vi "Add_TF_Ref.vi"(6 "TCP Ref":refnum<k5>, 8 "error in":errorcluster caption="错误输入", 10 "index":i32) -> (0 "error out":errorcluster caption="错误输出")   [LabVIEW 2015]
uses:
  Global/SeverGlobal.vi
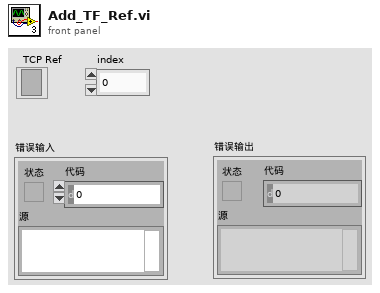
[diagram p1: front panel]
types:
  T1 = cluster{"TCP Ref":refnum<k5>, "Broadcast":refnum<k5>, "TF Ref":refnum<k5>, "IP":string, "port":u16, "userName":string, "passWord":string, "authority":string}[]
  T2 = cluster{"TCP Ref":refnum<k5>, "Broadcast":refnum<k5>, "TF":refnum<k5>, "IP":string, "port":u16, "userName":string, "passWord":string, "authority":string}
  T3 = cluster{"TCP Ref":refnum<k5>, "Broadcast":refnum<k5>, "TF Ref":refnum<k5>, "IP":string, "port":u16, "userName":string, "passWord":string, "authority":string}
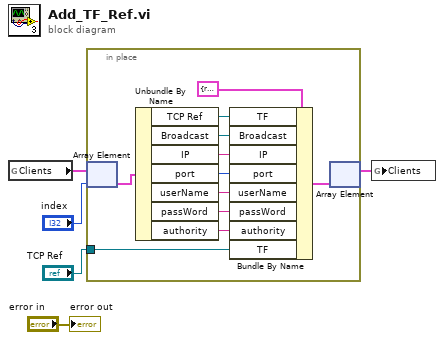
[diagram p0: block diagram]
diagram:
  n1 = global read "SeverGlobal.vi" "Clients"() -> (w4:T1)
  n2 = in-place {
    in-place-border: "TCP Ref" -> [w6]
    n3 = in-place-array #1(w4, "index") -> (w14:T3)
    n4 = Unbundle By Name(w14) -> ("TCP Ref"=w13:refnum<k5>, "Broadcast"=w12:refnum<k5>, "IP"=w11:string, "port"=w10:u16, "userName"=w9:string, "passWord"=w8:string, "authority"=w7:string)
    n5 = Bundle By Name(cluster=T2 {"TCP Ref"=refnum, "Broadcast"=refnum, "TF"=refnum, "IP"="", "port"=0, "userName"="", "passWord"="", "authority"=""} ("Client"), "TF"=w13, "Broadcast"=w12, "IP"=w11, "port"=w10, "userName"=w9, "passWord"=w8, "authority"=w7, "TF"=w6) -> (w15:T2)
    n6 = in-place-array #1(w15) -> (w1:T1)  [unwired: 1 out]
  }
  n7 = global write "SeverGlobal.vi" "Clients"(w1) -> ()
  "error out" <- "error in"
